vi "Access Type is null.vi"(8 "error in":errorcluster, 11 "Object Entry in":refnum<class "Object Entry.lvclass">) -> (0 "error out":errorcluster, 2 "Null":bool=TRUE, 3 "Object Entry out":refnum<class "Object Entry.lvclass">)   [LabVIEW 2020, in "CANopen.lvlib" / "Object Entry.lvclass"]
uses:
  Object Entry.lvclass
  Object Entry.lvclass/Object Entry.ctl
  Sub Object/Sub Object.lvclass
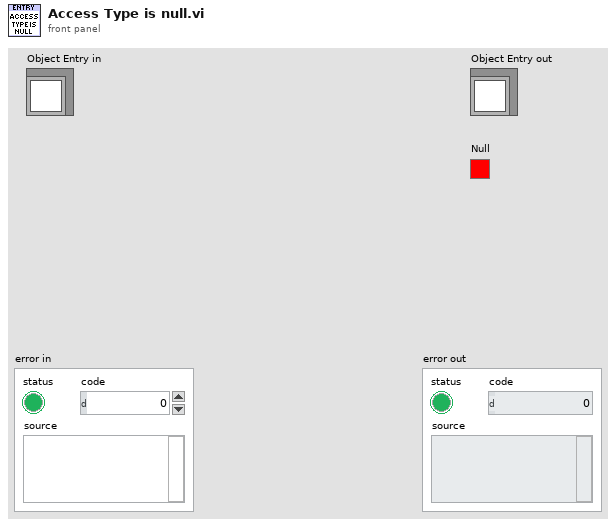
[diagram p1: front panel]
types:
  T1 = typedef "CANopen.lvlib/Object Type.ctl" = u8
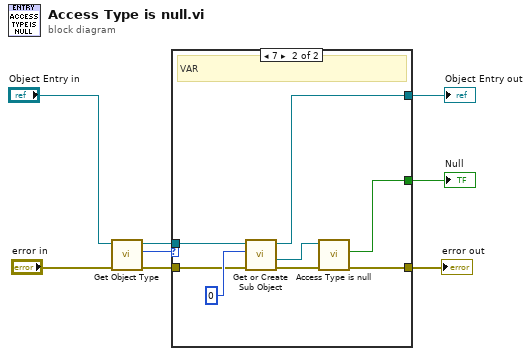
[diagram p0: block diagram]
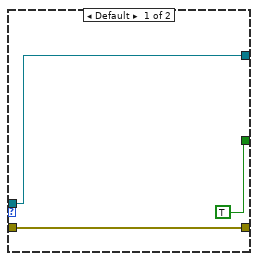
[diagram p2: hidden frame]
diagram:
  n1 = call "Get Object Type.vi"("error in"="error in", "Object Entry in"="Object Entry in") -> ("error out"=w6:errorcluster, "Object Type"=w3:T1, "Object Entry out"=w4:refnum<class "Object Entry.lvclass">)  [unwired: 7 in]
  n2 = case shown="7" w3 {
    tunnel: [w11 w17] -> w7
    tunnel: w6 -> [w11 w15]
    tunnel: w4 -> [w9 w14]
    tunnel: [TRUE ("Null") w13] -> w2
    tunnel: [w9 w12] -> w1
    frame Default {
    }
    frame 7 {
      # "VAR"
      n3 = call "Get or Create Sub Object.vi"("error in"=w15, "Sub Index"=u8 0, "Obj Entry in"=w14) -> ("error out"=w19:errorcluster, "Sub Object"=w16:refnum<class "Sub Object.lvclass">, "Obj Entry out"=w12:refnum<class "Object Entry.lvclass">)  [unwired: 6 in]
      n4 = call "Access Type is null.vi"("error in"=w19, "Sub Object in"=w16) -> ("error out"=w17:errorcluster, "Null"=w13:bool)  [unwired: 7 in, 1 out]
    }
  }
  "error out" <- w7
  "Object Entry out" <- w1
  "Null" <- w2
